vi "TDMS Report_Init.vi"(8 "error in (no error)":errorcluster) -> (0 "error out":errorcluster, 3 "TDMS Report out":refnum<class "Wind TDMS Report.lvclass">)   [LabVIEW 2009, in "Wind TDMS Report.lvclass"]
doc: "This creates a Wind TDMS Report object.\n\nAAL 9/09"
uses:
  Wind TDMS Report.lvclass
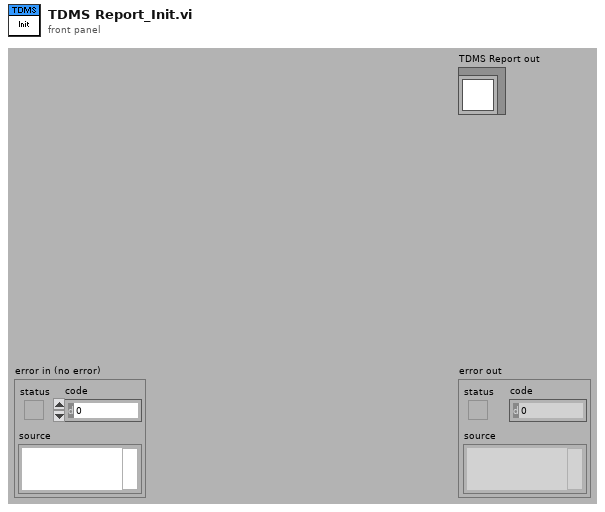
[diagram p1: front panel]
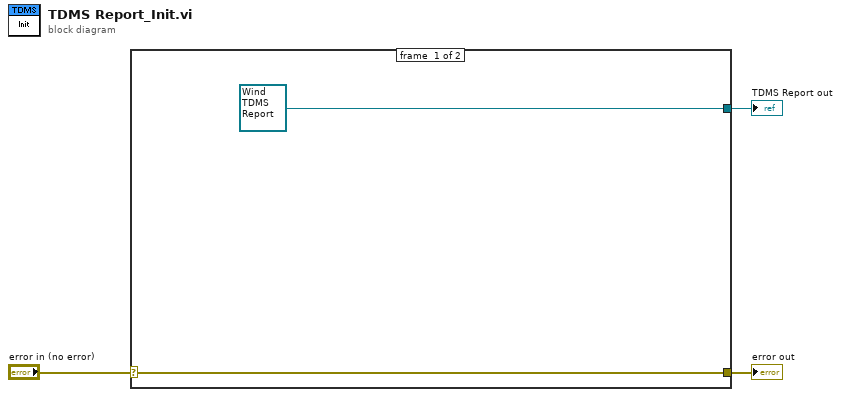
[diagram p0: block diagram]
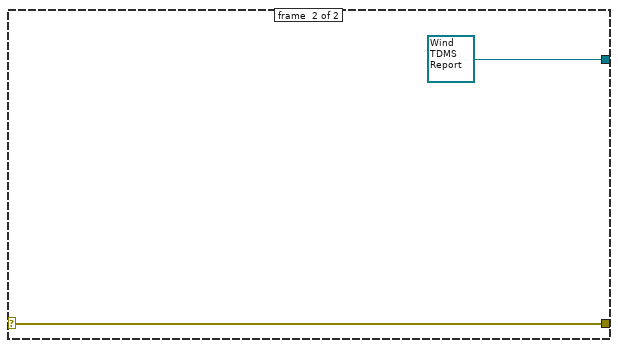
[diagram p2: hidden frame]
diagram:
  n1 = case shown="No Error" "error in (no error)" {
    selector: "error in (no error)" -> [w4 w7]
    tunnel: [w4 w7] -> w2
    tunnel: [refnum<class "Wind TDMS Report.lvclass"> refnum ("TXT_Report.lvclass") refnum<class "Wind TDMS Report.lvclass"> refnum ("TXT_Report.lvclass")] -> w1
    frame #0 {
    }
    frame #1 {
    }
  }
  "error out" <- w2
  "TDMS Report out" <- w1
